vi "Get Config File Name.vi"(8 "error in (no error)":errorcluster, 11 "Actor wUI in":refnum<class "Actor wUI.lvclass">) -> (0 "error out":errorcluster, 2 "Config File Name":string, 3 "Actor wUI out":refnum<class "Actor wUI.lvclass">)   [LabVIEW 2017, in "Framework.lvlib" / "Actor wUI.lvclass"]
uses:
  Actor wUI.lvclass
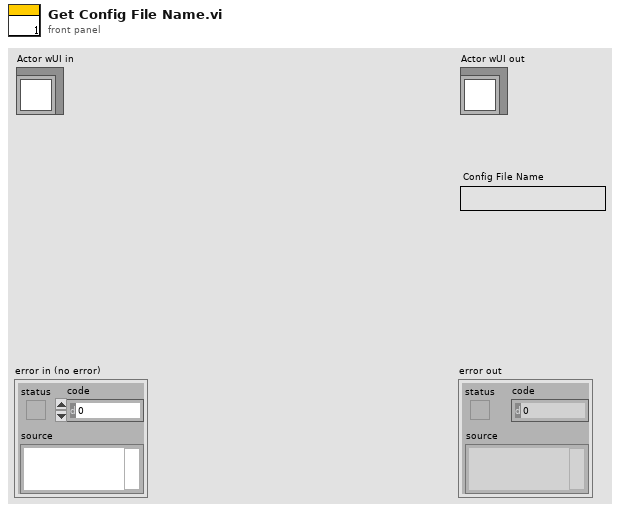
[diagram p1: front panel]
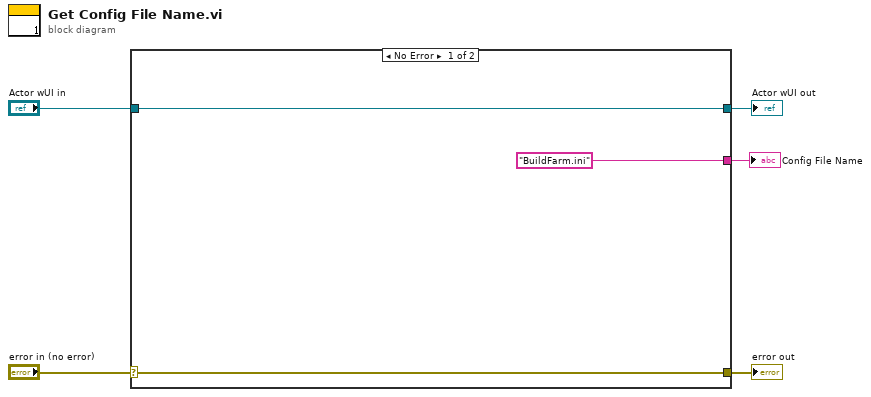
[diagram p0: block diagram]
diagram:
  n1 = case shown="No Error" "error in (no error)" {
    selector: "error in (no error)" -> [w7 w10]
    tunnel: [w7 w10] -> w4
    tunnel: [w8 w9] -> w2
    tunnel: "Actor wUI in" -> [w8 w9]
    tunnel: ["BuildFarm.ini" _] -> w1
    frame No Error {
    }
    frame Error {
    }
  }
  "error out" <- w4
  "Actor wUI out" <- w2
  "Config File Name" <- w1
